vi "Generate Index Array.vi"(1 "Size":i32) -> (0 "Index Array":dbl[](array[numeric]) format="%.2f")   [LabVIEW 2019]
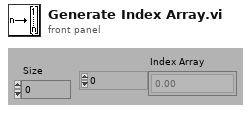
[diagram p1: front panel]
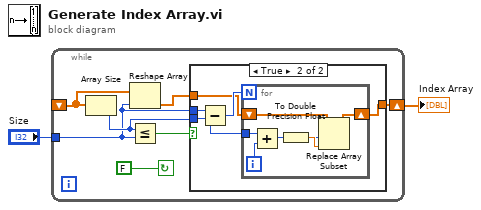
[diagram p0: block diagram]
diagram:
  n1 = while {
    tunnel: "Size" -> [w4]
    shift-left: _ -> [w8]
    shift-right: [w6] -> w1
    stop <- FALSE continue-if-true
    n2 = Array Size(array=w8) -> (size(s)=w5:i32)
    n3 = Reshape Array(w8, w4) -> (w7:dbl[])
    n4 = Less Or Equal?(x=w5, y=w4) -> (x <= y?=w9:bool)
    n5 = case shown="True" w9 {
      tunnel: w7 -> [w10 w12]
      tunnel: [w10 w11] -> w6
      tunnel: w5 -> [_ w15]
      tunnel: w4 -> [_ w14]
      frame False {
      }
      frame True {
        n6 = Subtract(x=w14, y=w15) -> (x-y=w13:i32)
        n7 = for {
          N: w13 -> [_]
          tunnel: w15 -> [w20]
          shift-right: [w16] -> w11
          shift-left: w12 -> [w17]
          i -> [w21]
          n8 = Add(x=w20, y=w21) -> (x+y=w18:i32)
          n9 = To Double Precision Float(number=w18) -> (double precision float=w19:dbl)
          n10 = Replace Array Subset(array=w17, new element=w19, index=w18) -> (w16:dbl[])
        }
      }
    }
  }
  "Index Array" <- w1
